vi "get supported types.vi"(8 "error in":errorcluster, 11 "module configuration in":refnum<class "TBM module configuration.lvclass">) -> (0 "error out":errorcluster, 2 "supported types":T1[](array[typedef]), 3 "module configuration out":refnum<class "TBM module configuration.lvclass">)   [LabVIEW 2014, in "TBM module configuration.lvclass"]
doc: "Provides an interface for determining the targets supported by a given configuration/runtime class pairing. This should be overridden by any useful child class."
uses:
  TBM module configuration.lvclass
  <vilib>/NI/Tag Bus/tag/Data Type.ctl
  <vilib>/NI/Tag Bus/tag/tag descriptor.lvclass
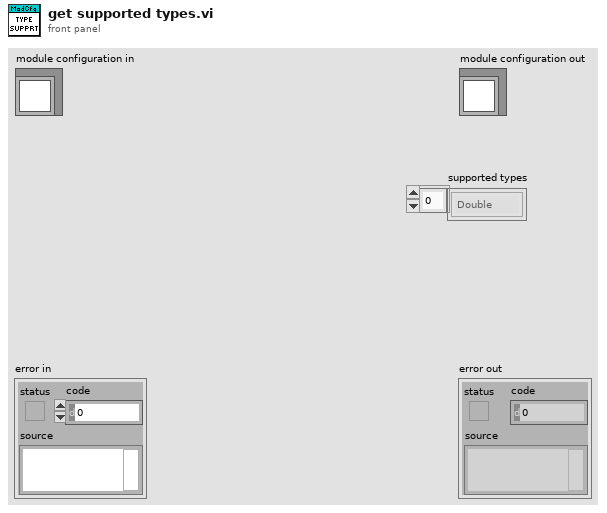
[diagram p1: front panel]
types:
  T1 = typedef "tag bus.lvlib/tag descriptor.lvclass/Data Type.ctl" = enum16{"Double", "Single", "I64", "I32", "I16", "I8", "U64", "U32", "U16", "U8", "Boolean", "String", "Array of Double", "Array of Single", "Array of I64", "Array of I32", "Array of I16", "Array of I8", "Array of U64", "Array of U32", "Array of U16", "Array of U8", "Array of Boolean", "Array of String"}
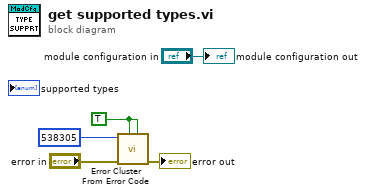
[diagram p0: block diagram]
diagram:
  w3 = TRUE ("is warning? (False)")
  n1 = call <vilib>:"Error Cluster From Error Code.vi"("is warning? (False)"=w3, "show call chain? (False)"=w3, "error in (no error)"="error in", "error code (0)"=538305) -> ("error out"=→"error out":errorcluster)  [unwired: 5 in]
  "module configuration out" <- "module configuration in"
